vi "Init.vi"(8 "error in":errorcluster, 10 "<JSON> Scaling Config":string, 11 "Linear Scaling Strategy in":refnum<class "Linear Scaling Strategy.lvclass">) -> (0 "error out":errorcluster, 3 "Linear Scaling Strategy out":refnum<class "Linear Scaling Strategy.lvclass">)   [LabVIEW 2024, in "HAL.lvlib" / "Linear Scaling Strategy.lvclass"]
uses:
  Linear Scaling Strategy.lvclass
  Linear Scaling Strategy.lvclass/Linear Scaling Strategy.ctl
  143502c1-08e5-457a-9666-ae3b3c0b3bd1.vi
  <vilib>/JDP Science/JSONtext/JSON text to Variant.vi
  <vilib>/JDP Science/JSONtext/LVClass Serializer/JSONtext LVClass Serializer.lvclass
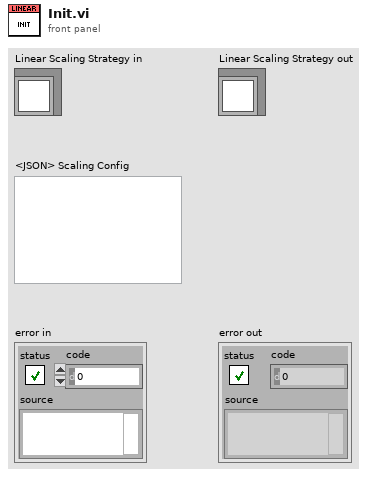
[diagram p1: front panel]
types:
  T1 = cluster{"Input min":dbl, "Output min":dbl, "Input max":dbl, "Output max":dbl}
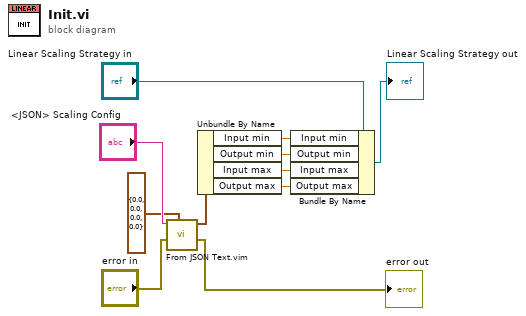
[diagram p0: block diagram]
diagram:
  n1 = call "From JSON Text.vim"("Data Type and Default Value"=T1 {"Input min"=0.0, "Output min"=0.0, "Input max"=0.0, "Output max"=0.0}, "error in (no error)"="error in", "JSON"="<JSON> Scaling Config") -> ("error out"=→"error out":errorcluster, "Data out"=w6:T1)  [unwired: 7 in]
  n2 = Unbundle By Name(w6) -> ("Input min"=w5:dbl, "Output min"=w4:dbl, "Input max"=w3:dbl, "Output max"=w2:dbl)
  n3 = Bundle By Name(cluster="Linear Scaling Strategy in", "Input min"=w5, "Output min"=w4, "Input max"=w3, "Output max"=w2) -> (→"Linear Scaling Strategy out":refnum<class "Linear Scaling Strategy.lvclass">)
